vi "FitFunction.vi"(3 "output control":T1, 4 "data":T2, 5 "X":dbl[](array[numeric]), 6 "a":dbl[](array[numeric])) -> (0 "error out":errorcluster, 1 "f'(X,a)":dbl[][](array[numeric]), 2 "f(X,a)(G)":dbl[](array[numeric]))   [LabVIEW 2012]
doc: "This template is the starting point for creating a model function to be passed to the Nonlinear Curve Fit.vi."
uses:
  <vilib>/gmath/NumericalOptimization/objective function data.ctl
  <vilib>/gmath/NumericalOptimization/LM_output select.ctl
  <vilib>/gmath/NI_Gmath.lvlib
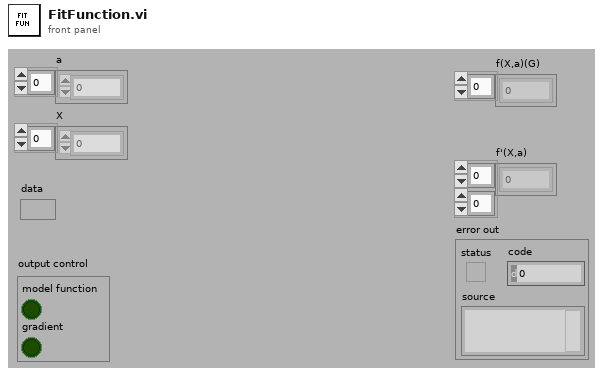
[diagram p1: front panel]
types:
  T1 = typedef "NI_Gmath.lvlib/LM_output select.ctl" = cluster{"model function":bool, "gradient":bool}
  T2 = typedef "NI_Gmath.lvlib/objective function data.ctl" = variant
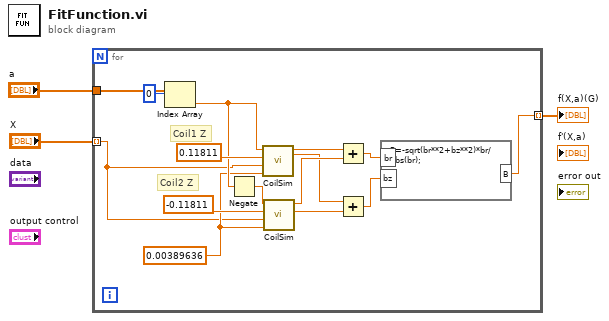
[diagram p0: block diagram]
diagram:
  n1 = for {
    tunnel: "X" -> [w4] mode=indexing
    tunnel: [w9] -> w2 mode=indexing
    tunnel: "a" -> [w6]
    w7 = 0.00389636 ("z(m)")
    # "Coil2 Z"
    # "Coil1 Z"
    n2 = Index Array(array=w6, index=0) -> (element=w8:dbl)
    n3 = Negate(x=w8) -> (-x=w16:dbl)
    n4 = call "CoilSim.vi"("z(m)"=w7, "x(m)"=w4, "zp(m)"=0.11811, "I(A)"=w8) -> ("Bz(G)"=w13:dbl, "Br(G)"=w15:dbl)  [unwired: 6 in]
    n5 = call "CoilSim.vi"("z(m)"=w7, "x(m)"=w4, "zp(m)"=-0.11811, "I(A)"=w16) -> ("Bz(G)"=w12:dbl, "Br(G)"=w14:dbl)  [unwired: 6 in]
    n6 = Add(x=w15, y=w14) -> (x+y=w11:dbl)
    n7 = Add(x=w13, y=w12) -> (x+y=w10:dbl)
    n8 = formula code="B=-sqrt(br**2+bz**2)*br/abs(br);"("br"=w11, "bz"=w10) -> ("B"=w9:dbl)
  }
  "f(X,a)(G)" <- w2
